vi "FGV_DLL Action.vi"(7 "State":enum16{"Initial", "Run", "Close"}(ring), 8 "Error In":errorcluster, 9 "Model Index":i32, 11 "Project name":string) -> (0 "Error Out":errorcluster)   [LabVIEW 2015]
uses:
  <vilib>/Utility/xml.llb/Read From XML File(string).vi
  <vilib>/measure/NI_MABase.lvlib
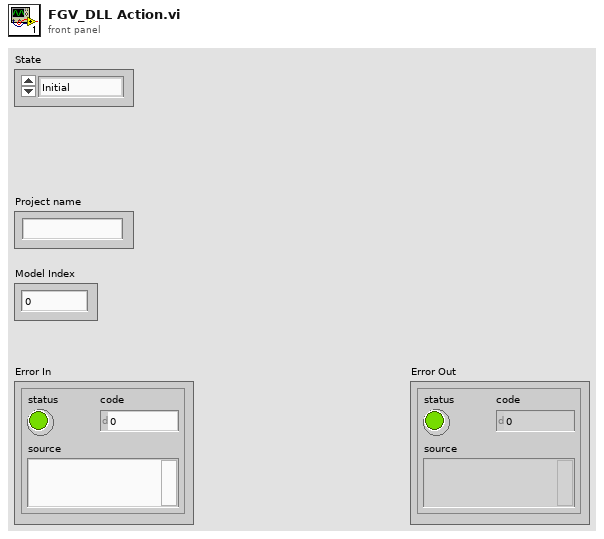
[diagram p1: front panel]
types:
  T1 = cluster{"Channel 1":cluster{" frequency 1":i32, "signal type 1":enum16{"Sine Wave", "Triangle Wave", "Square Wave", "Sawtooth Wave"}, "amplitude 1":dbl, "offset":i32, "phase":dbl}, "Channel 2":cluster{" frequency 1":i32, "signal type 1":enum16{"Sine Wave", "Triangle Wave", "Square Wave", "Sawtooth Wave"}, "amplitude 1":dbl, "offset":i32, "phase":i32}, "Channel 3":cluster{" frequency 1":i32, "signal type 1":enum16{"Sine Wave", "Triangle Wave", "Square Wave", "Sawtooth Wave"}, "amplitude 1":dbl, "offset":i32, "phase":i32}, "Channel 4":cluster{" frequency 1":i32, "signal type 1":enum16{"Sine Wave", "Triangle Wave", "Square Wave", "Sawtooth Wave"}, "amplitude 1":dbl, "offset":i32, "phase":i32}}
  T2 = cluster{" frequency 1":i32, "signal type 1":enum16{"Sine Wave", "Triangle Wave", "Square Wave", "Sawtooth Wave"}, "amplitude 1":dbl, "offset":i32, "phase":dbl}
  T3 = cluster{" frequency 1":i32, "signal type 1":enum16{"Sine Wave", "Triangle Wave", "Square Wave", "Sawtooth Wave"}, "amplitude 1":dbl, "offset":i32, "phase":i32}
  T4 = cluster{" frequency 1":i32, "signal type 1":enum16{"Sine Wave", "Triangle Wave", "Square Wave", "Sawtooth Wave"}, "amplitude 1":dbl, "offset":i32, "phase":dbl}[]
  T5 = enum16{"Sine Wave", "Triangle Wave", "Square Wave", "Sawtooth Wave"}
  T6 = cluster{"Channel 1":cluster{" frequency 1":u32, "signal type 1":enum16{"Sine Wave", "Triangle Wave", "Square Wave", "Sawtooth Wave"}, "amplitude 1":dbl, "offset":dbl, "phase":dbl}, "Channel 2":cluster{" frequency 1":u32, "signal type 1":enum16{"Sine Wave", "Triangle Wave", "Square Wave", "Sawtooth Wave"}, "amplitude 1":dbl, "offset":dbl, "phase":dbl}, "Channel 3":cluster{" frequency 1":u32, "signal type 1":enum16{"Sine Wave", "Triangle Wave", "Square Wave", "Sawtooth Wave"}, "amplitude 1":dbl, "offset":dbl, "phase":dbl}, "Channel 4":cluster{" frequency 1":u32, "signal type 1":enum16{"Sine Wave", "Triangle Wave", "Square Wave", "Sawtooth Wave"}, "amplitude 1":dbl, "offset":dbl, "phase":dbl}, "Time(ms)":i32, "Rate":dbl, "Channel 1 Sample":cluster{"Sample Rate":dbl, "Samples":dbl}, "Channel 2 Sample":cluster{"Sample Rate":dbl, "Samples":dbl}, "Channel 3 Sample":cluster{"Sample Rate":dbl, "Samples":dbl}, "Channel 4 Sample":cluster{"Sample Rate":dbl, "Samples":dbl}}[]
  T7 = cluster{"DAQ name":string, "DataTable":cluster{"Channel 1":cluster{" frequency 1":u32, "signal type 1":enum16{"Sine Wave", "Triangle Wave", "Square Wave", "Sawtooth Wave"}, "amplitude 1":dbl, "offset":dbl, "phase":dbl}, "Channel 2":cluster{" frequency 1":u32, "signal type 1":enum16{"Sine Wave", "Triangle Wave", "Square Wave", "Sawtooth Wave"}, "amplitude 1":dbl, "offset":dbl, "phase":dbl}, "Channel 3":cluster{" frequency 1":u32, "signal type 1":enum16{"Sine Wave", "Triangle Wave", "Square Wave", "Sawtooth Wave"}, "amplitude 1":dbl, "offset":dbl, "phase":dbl}, "Channel 4":cluster{" frequency 1":u32, "signal type 1":enum16{"Sine Wave", "Triangle Wave", "Square Wave", "Sawtooth Wave"}, "amplitude 1":dbl, "offset":dbl, "phase":dbl}, "Time(ms)":i32, "Rate":dbl, "Channel 1 Sample":cluster{"Sample Rate":dbl, "Samples":dbl}, "Channel 2 Sample":cluster{"Sample Rate":dbl, "Samples":dbl}, "Channel 3 Sample":cluster{"Sample Rate":dbl, "Samples":dbl}, "Channel 4 Sample":cluster{"Sample Rate":dbl, "Samples":dbl}}[], "Item Names":string[]}
  T8 = cluster{"DataTable":cluster{"Channel 1":cluster{" frequency 1":u32, "signal type 1":enum16{"Sine Wave", "Triangle Wave", "Square Wave", "Sawtooth Wave"}, "amplitude 1":dbl, "offset":dbl, "phase":dbl}, "Channel 2":cluster{" frequency 1":u32, "signal type 1":enum16{"Sine Wave", "Triangle Wave", "Square Wave", "Sawtooth Wave"}, "amplitude 1":dbl, "offset":dbl, "phase":dbl}, "Channel 3":cluster{" frequency 1":u32, "signal type 1":enum16{"Sine Wave", "Triangle Wave", "Square Wave", "Sawtooth Wave"}, "amplitude 1":dbl, "offset":dbl, "phase":dbl}, "Channel 4":cluster{" frequency 1":u32, "signal type 1":enum16{"Sine Wave", "Triangle Wave", "Square Wave", "Sawtooth Wave"}, "amplitude 1":dbl, "offset":dbl, "phase":dbl}, "Time(ms)":i32, "Rate":dbl, "Channel 1 Sample":cluster{"Sample Rate":dbl, "Samples":dbl}, "Channel 2 Sample":cluster{"Sample Rate":dbl, "Samples":dbl}, "Channel 3 Sample":cluster{"Sample Rate":dbl, "Samples":dbl}, "Channel 4 Sample":cluster{"Sample Rate":dbl, "Samples":dbl}}[], "Item Names":string[]}
  T9 = cluster{"Channel 1":cluster{" frequency 1":u32, "signal type 1":enum16{"Sine Wave", "Triangle Wave", "Square Wave", "Sawtooth Wave"}, "amplitude 1":dbl, "offset":dbl, "phase":dbl}, "Channel 2":cluster{" frequency 1":u32, "signal type 1":enum16{"Sine Wave", "Triangle Wave", "Square Wave", "Sawtooth Wave"}, "amplitude 1":dbl, "offset":dbl, "phase":dbl}, "Channel 3":cluster{" frequency 1":u32, "signal type 1":enum16{"Sine Wave", "Triangle Wave", "Square Wave", "Sawtooth Wave"}, "amplitude 1":dbl, "offset":dbl, "phase":dbl}, "Channel 4":cluster{" frequency 1":u32, "signal type 1":enum16{"Sine Wave", "Triangle Wave", "Square Wave", "Sawtooth Wave"}, "amplitude 1":dbl, "offset":dbl, "phase":dbl}, "Time(ms)":i32, "Rate":dbl, "Channel 1 Sample":cluster{"Sample Rate":dbl, "Samples":dbl}, "Channel 2 Sample":cluster{"Sample Rate":dbl, "Samples":dbl}, "Channel 3 Sample":cluster{"Sample Rate":dbl, "Samples":dbl}, "Channel 4 Sample":cluster{"Sample Rate":dbl, "Samples":dbl}}
  T10 = cluster{" frequency 1":u32, "signal type 1":enum16{"Sine Wave", "Triangle Wave", "Square Wave", "Sawtooth Wave"}, "amplitude 1":dbl, "offset":dbl, "phase":dbl}
  T11 = cluster{" frequency 1":u32, "signal type 1":enum16{"Sine Wave", "Triangle Wave", "Square Wave", "Sawtooth Wave"}, "amplitude 1":dbl, "offset":dbl, "phase":dbl}[]
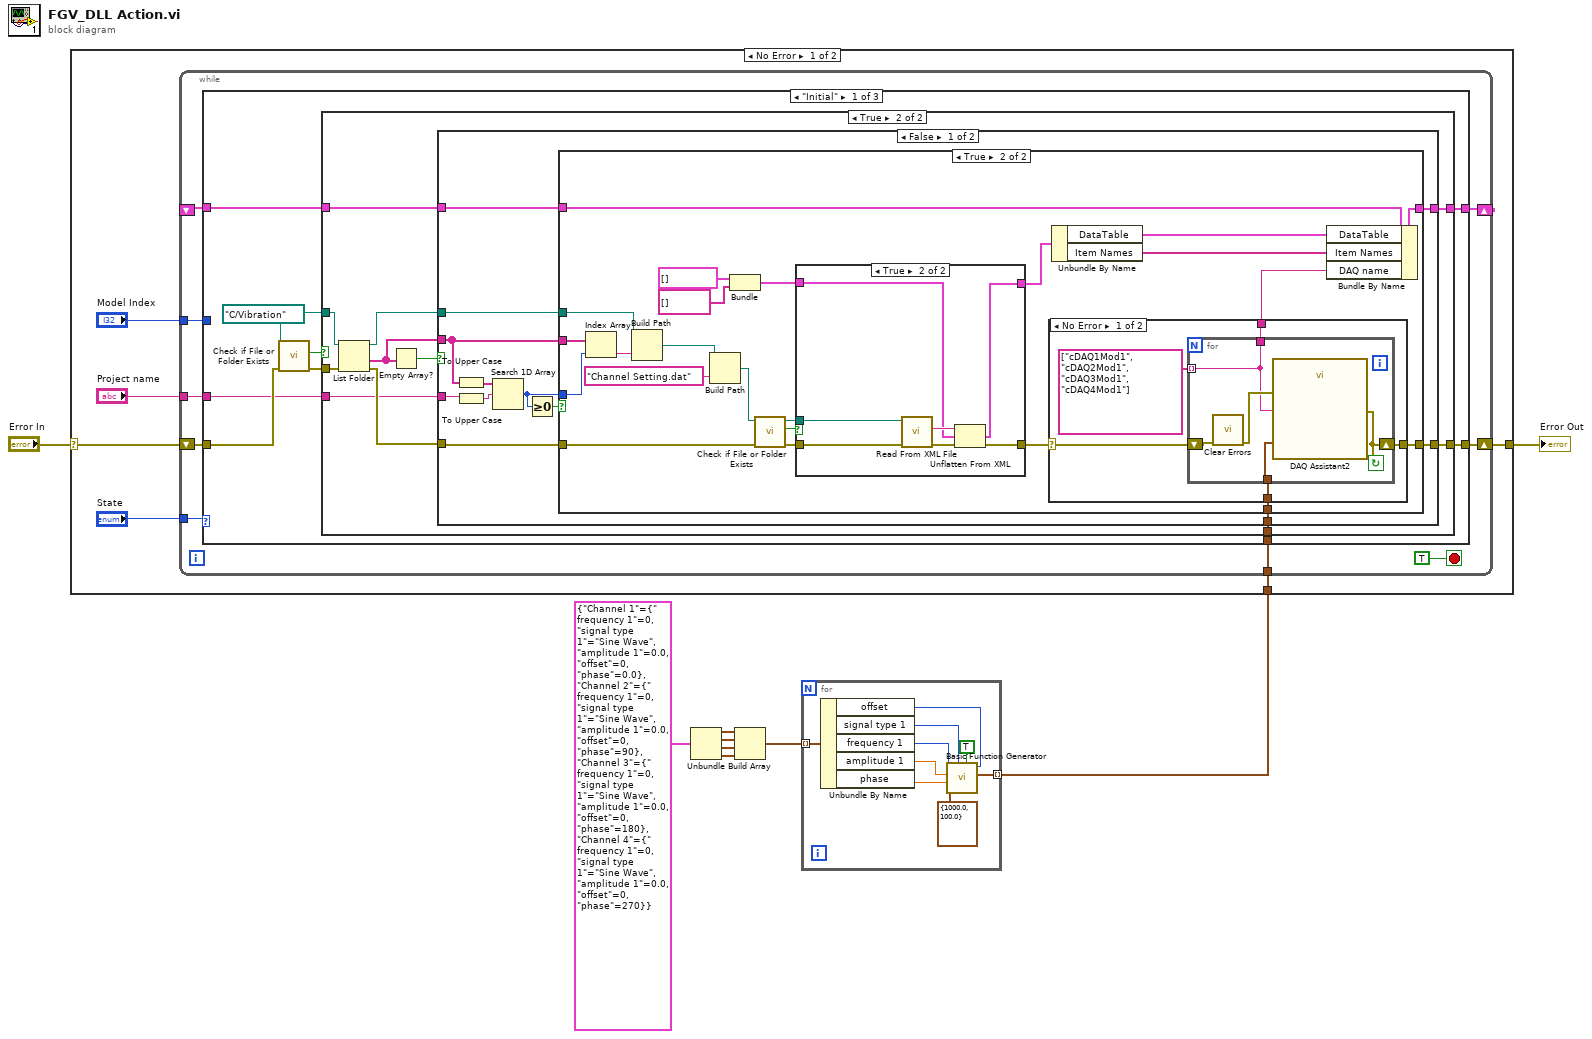
[diagram p0: block diagram]
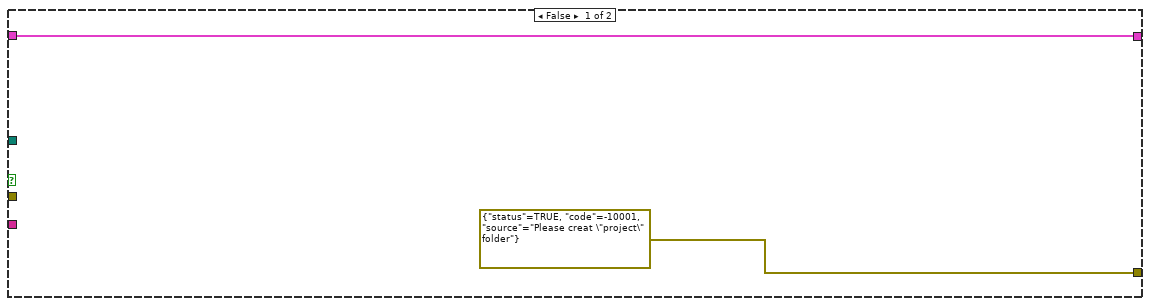
[diagram p2: hidden frame]
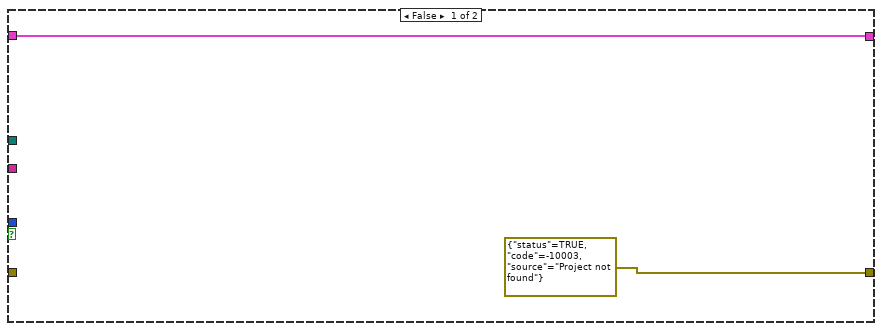
[diagram p3: hidden frame]
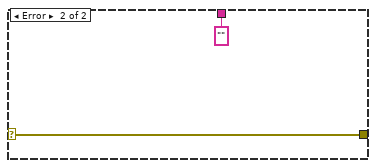
[diagram p4: hidden frame]
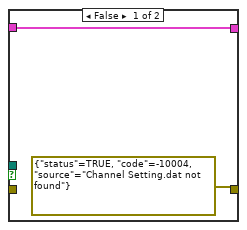
[diagram p5: hidden frame]
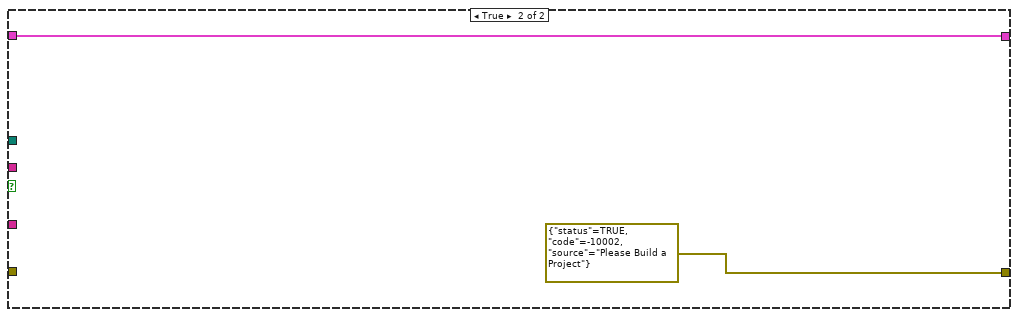
[diagram p6: hidden frame]
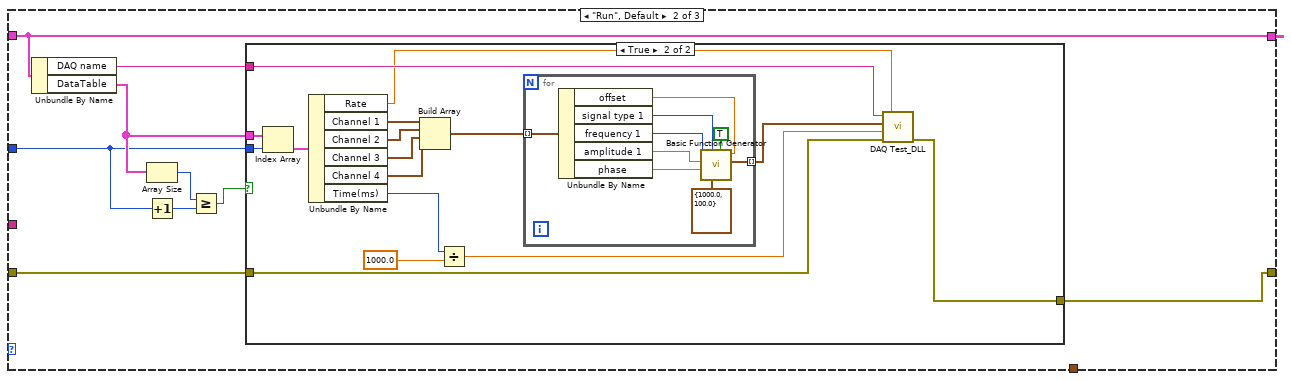
[diagram p7: hidden frame]
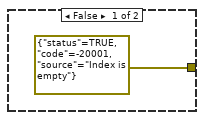
[diagram p8: hidden frame]
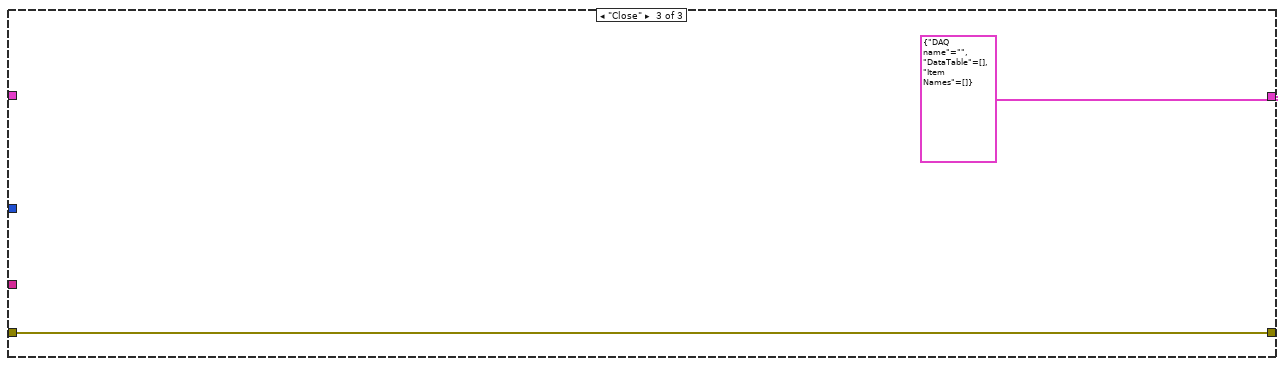
[diagram p9: hidden frame]
diagram:
  n1 = Unbundle(T1 {"Channel 1"={" frequency 1"=0, "signal type 1"=enum."Sine Wave", "amplitude 1"=0.0, "offset"=0, "phase"=0.0}, "Channel 2"={" frequency 1"=0, "signal type 1"=enum."Sine Wave", "amplitude 1"=0.0, "offset"=0, "phase"=90}, "Channel 3"={" frequency 1"=0, "signal type 1"=enum."Sine Wave", "amplitude 1"=0.0, "offset"=0, "phase"=180}, "Channel 4"={" frequency 1"=0, "signal type 1"=enum."Sine Wave", "amplitude 1"=0.0, "offset"=0, "phase"=270}} ("Center")) -> ("Channel 1"=w7:T2, "Channel 2"=w6:T3, "Channel 3"=w5:T3, "Channel 4"=w4:T3)
  n2 = Build Array(w7, w6, w5, w4) -> (w3:T4)
  n3 = for {
    tunnel: w3 -> [w10] mode=indexing
    tunnel: [w11] -> w2 mode=indexing
    n4 = Unbundle By Name(w10) -> ("offset"=w12:i32, "signal type 1"=w13:T5, "frequency 1"=w14:i32, "amplitude 1"=w15:dbl, "phase"=w16:dbl)
    n5 = call <vilib>:"Basic Function Generator.vi"("offset"=w12, "reset signal"=TRUE, "sampling info"=cluster{"Fs":dbl, "#s":dbl} {"Fs"=1000.0, "#s"=100.0} ("sampling info 4"), "signal type"=w13, "phase"=w16, "amplitude"=w15, "frequency"=w14) -> ("signal out"=w11:waveform(dbl))  [unwired: 2 in, 2 out]
  }
  n6 = case shown="No Error" "Error In" {
    selector: "Error In" -> [w23 w153]
    tunnel: [w22 w153] -> w8
    tunnel: w2 -> [w19 _]
    frame No Error {
      n7 = while {
        tunnel: "State" -> [w33]
        shift-right: [w31] -> w22
        shift-left: w23 -> [w32]
        shift-right: [w29] -> _
        shift-left: _ -> [w30]
        tunnel: "Project name" -> [w28]
        tunnel: "Model Index" -> [w26]
        tunnel: w19 -> [w25]
        stop <- TRUE stop-if-true
        n8 = case shown="\"Initial\"" w33 {
          tunnel: w32 -> [w40 w122 w152]
          tunnel: [w42 w121 w152] -> w31
          tunnel: w30 -> [w37 w123 _]
          tunnel: [w36 w123 T7 {"DAQ name"="", "DataTable"=[], "Item Names"=[]}] -> w29
          tunnel: w28 -> [w35 _ _]
          tunnel: w26 -> [_ w119 _]
          tunnel: w25 -> [w34 _ _]
          frame "Initial" {
            w41 = path "C:/Vibration"
            n9 = call <vilib>:"Check if File or Folder Exists.vi"("error in (no error)"=w40, "path"=w41) -> ("error out"=w39:errorcluster, "file or folder exists?"=w38:bool)  [unwired: 7 in, 1 out]
            n10 = case shown="True" w38 {
              tunnel: [errorcluster {"status"=TRUE, "code"=-10001, "source"="Please creat \"project\" folder"} ("error out") w53] -> w42
              tunnel: w41 -> [_ w47]
              tunnel: w39 -> [_ w52]
              tunnel: w37 -> [w44 w51]
              tunnel: [w44 w50] -> w36
              tunnel: w35 -> [_ w49]
              tunnel: w34 -> [_ w45]
              frame False {
              }
              frame True {
                n11 = List Folder(path=w47, error in=w52) -> (path out=w46:path, folder names=w48:string[], error out=w54:errorcluster)  [unwired: 2 in, 1 out]
                n12 = Empty Array?(array=w48) -> (empty?=w55:bool)
                n13 = case shown="False" w55 {
                  tunnel: w54 -> [w65 _]
                  tunnel: w46 -> [w63 _]
                  tunnel: [w64 errorcluster {"status"=TRUE, "code"=-10002, "source"="Please Build a Project"} ("error out")] -> w53
                  tunnel: w51 -> [w67 w115]
                  tunnel: [w66 w115] -> w50
                  tunnel: w49 -> [w61 _]
                  tunnel: w48 -> [w59 _]
                  tunnel: w45 -> [w56 _]
                  frame False {
                    n14 = To Upper Case(1:w59) -> (0:w62:string[])
                    n15 = To Upper Case(1:w61) -> (0:w60:string)
                    n16 = Search 1D Array(1D array=w62, element=w60) -> (index of element=w58:i32)  [unwired: 1 in]
                    n17 = Greater Or Equal To 0?(x=w58) -> (x >= 0?=w57:bool)
                    n18 = case shown="True" w57 {
                      tunnel: w67 -> [w69 w92]
                      tunnel: [w69 w91] -> w66
                      tunnel: w65 -> [_ w76]
                      tunnel: [errorcluster {"status"=TRUE, "code"=-10003, "source"="Project not found"} ("error out") w72] -> w64
                      tunnel: w63 -> [_ w84]
                      tunnel: w59 -> [_ w81]
                      tunnel: w58 -> [_ w80]
                      tunnel: w56 -> [_ w71]
                      frame False {
                      }
                      frame True {
                        n19 = Index Array(array=w81, index=w80) -> (element=w79:string)
                        n20 = Build Path(base path=w84, name or relative path=w79) -> (appended path=w83:path)
                        n21 = Build Path(base path=w83, name or relative path="Channel Setting.dat") -> (appended path=w78:path)
                        n22 = Bundle("DataTable"=T6 [], "Item Names"=string[] []) -> (w88:T8)  [unwired: 1 in]
                        n23 = call <vilib>:"Check if File or Folder Exists.vi"("error in (no error)"=w76, "path"=w78) -> ("error out"=w75:errorcluster, "file or folder exists?"=w77:bool, "dup path"=w74:path)  [unwired: 7 in]
                        n24 = case shown="True" w77 {
                          tunnel: w75 -> [_ w113]
                          tunnel: w88 -> [w106 w110]
                          tunnel: [errorcluster {"status"=TRUE, "code"=-10004, "source"="Channel Setting.dat not found"} ("error out") w109] -> w73
                          tunnel: [w106 w108] -> w87
                          tunnel: w74 -> [_ w107]
                          frame False {
                          }
                          frame True {
                            n25 = call-poly <vilib>:"Read From XML File.vi"("error in (no error)"=w113, "XML File Path"=w107) -> ("error out"=w111:errorcluster, "XML Elements"=w112:string)  [unwired: 7 in, 1 out]
                            n26 = Unflatten From XML(xml string=w112, type=w110, error in (no error)=w111) -> (value=w108:T8, error out=w109:errorcluster)
                          }
                        }
                        n27 = case shown="No Error" w73 {
                          selector: w73 -> [w97 w104]
                          tunnel: [w96 w104] -> w72
                          tunnel: w71 -> [w95 _]
                          tunnel: [w93 ""] -> w70
                          frame No Error {
                            n28 = for {
                              tunnel: w95 -> [w101]
                              shift-right: [w100] -> w96
                              shift-left: w97 -> [w102]
                              tunnel: string[] ["cDAQ1Mod1", "cDAQ2Mod1", "cDAQ3Mod1", "cDAQ4Mod1"] -> [w98] mode=indexing
                              tunnel: [w98] -> w93
                              stop <- w100 continue-if-true
                              n29 = call <vilib>:"Clear Errors.vi"("error in (no error)"=w102) -> ("error out"=w99:errorcluster)  [unwired: 5 in, 1 out]
                              n30 = call "DAQ Assistant2"("data"=w101, "error in"=w99, "device name"=w98) -> ("error out"=w100:errorcluster)  [unwired: 15 in, 1 out]
                            }
                          }
                          frame Error {
                          }
                        }
                        n31 = Unbundle By Name(w87) -> ("DataTable"=w86:T6, "Item Names"=w85:string[])
                        n32 = Bundle By Name(cluster=w92, "DataTable"=w86, "Item Names"=w85, "DAQ name"=w70) -> (w91:T7)
                      }
                    }
                  }
                  frame True {
                  }
                }
              }
            }
          }
          frame "Run", Default {
            n33 = Unbundle By Name(w123) -> ("DAQ name"=w124:string, "DataTable"=w120:T6)
            n34 = Array Size(array=w120) -> (size(s)=w117:i32)
            n35 = Increment(x=w119) -> (x+1=w118:i32)
            n36 = Greater Or Equal?(x=w117, y=w118) -> (x >= y?=w116:bool)
            n37 = case shown="True" w116 {
              tunnel: w120 -> [_ w137]
              tunnel: w124 -> [_ w132]
              tunnel: w122 -> [_ w133]
              tunnel: w119 -> [_ w136]
              tunnel: [errorcluster {"status"=TRUE, "code"=-20001, "source"="Index is empty"} ("t") w129] -> w121
              frame False {
              }
              frame True {
                n38 = Index Array(array=w137, index=w136) -> (element=w135:T9)
                n39 = Unbundle By Name(w135) -> ("Rate"=w130:dbl, "Channel 1"=w141:T10, "Channel 2"=w140:T10, "Channel 3"=w139:T10, "Channel 4"=w138:T10, "Time(ms)"=w128:i32)
                n40 = Build Array(w141, w140, w139, w138) -> (w134:T11)
                n41 = Divide(x=w128, y=1000.0) -> (x/y=w126:dbl)
                n42 = for {
                  tunnel: [w143] -> w131 mode=indexing
                  tunnel: w134 -> [w142] mode=indexing
                  n43 = Unbundle By Name(w142) -> ("offset"=w144:dbl, "signal type 1"=w145:T5, "frequency 1"=w146:u32, "amplitude 1"=w147:dbl, "phase"=w148:dbl)
                  n44 = call <vilib>:"Basic Function Generator.vi"("offset"=w144, "reset signal"=TRUE, "sampling info"=cluster{"Fs":dbl, "#s":dbl} {"Fs"=1000.0, "#s"=100.0} ("sampling info 4"), "signal type"=w145, "phase"=w148, "amplitude"=w147, "frequency"=w146) -> ("signal out"=w143:waveform(dbl))  [unwired: 2 in, 2 out]
                }
                n45 = call "DAQ Test_DLL.vi"("rate"=w130, "error in"=w133, "Time"=w126, "data"=w131, "device name"=w132) -> ("error out"=w129:errorcluster)  [unwired: 5 in, 1 out]
              }
            }
          }
          frame "Close" {
          }
        }
      }
    }
    frame Error {
    }
  }
  "Error Out" <- w8
